vi "Property Finder (SubVI).vi"(8 "error in (no error)":errorcluster, 10 "Enum":enum16{"Read File", "Search for Property Name"}(ring), 11 "Property Name":string) -> (0 "error out":errorcluster, 3 "Property Value":string)   [LabVIEW 2018]
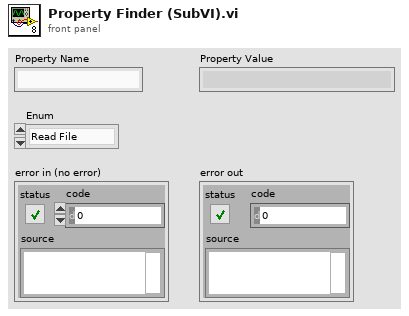
[diagram p1: front panel]
types:
  T1 = enum16{"open", "replace", "create", "open or create", "replace or create", "replace or create with confirmation"}
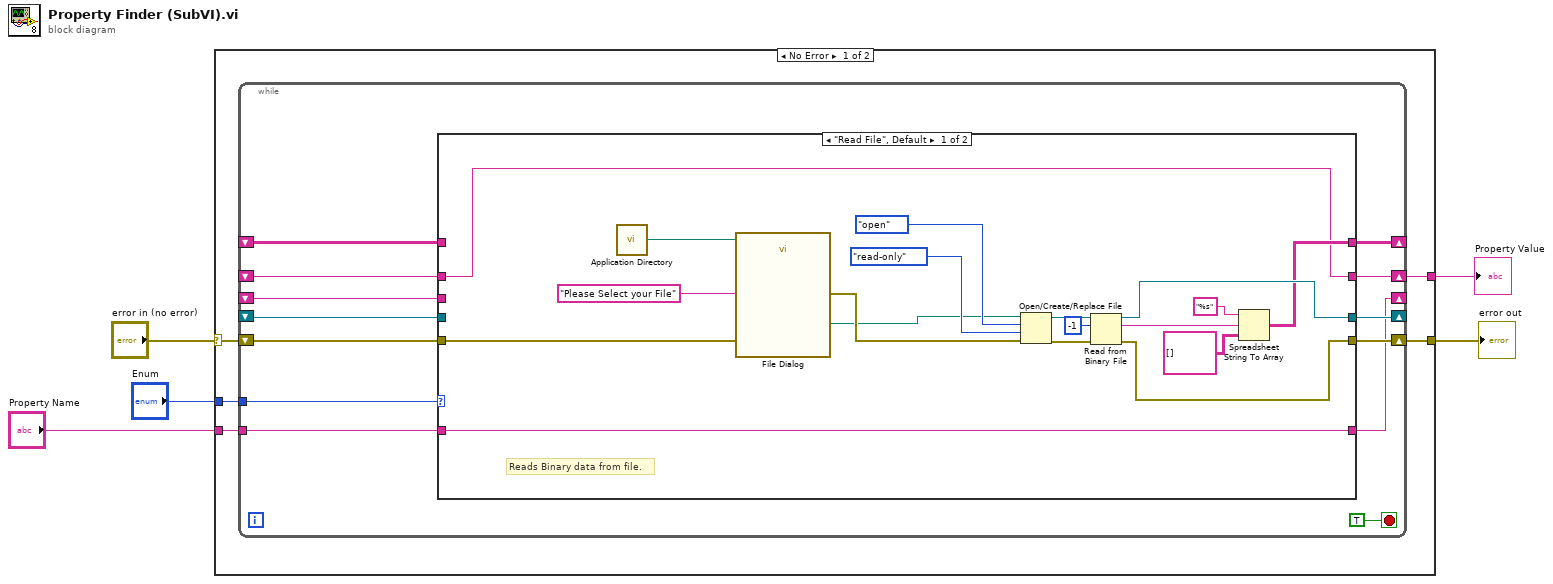
[diagram p0: block diagram]
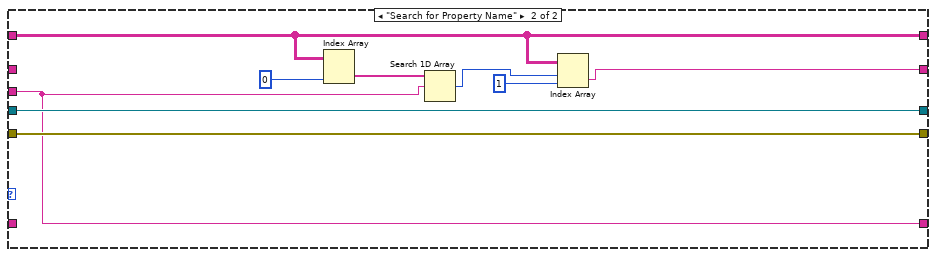
[diagram p2: hidden frame]
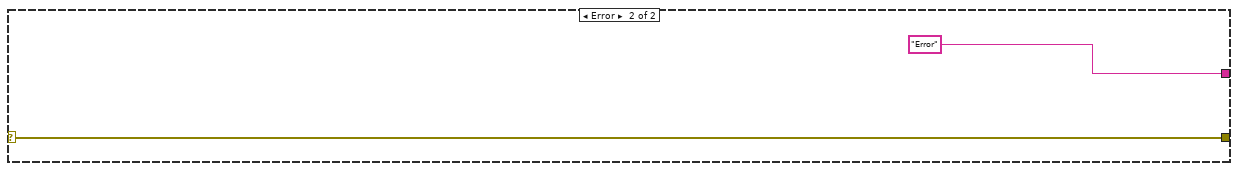
[diagram p3: hidden frame]
diagram:
  n1 = case shown="No Error" "error in (no error)" {
    selector: "error in (no error)" -> [w8 w52]
    tunnel: "Enum" -> [w10 _]
    tunnel: [w9 w52] -> w2
    tunnel: "Property Name" -> [w6 _]
    tunnel: [w7 "Error"] -> w5
    frame No Error {
      n2 = while {
        tunnel: w10 -> [w23]
        shift-right: [w21] -> w9
        shift-left: w8 -> [w20]
        shift-right: [w19] -> _
        shift-left: _ -> [w18]
        shift-right: [w16] -> _
        shift-left: _ -> [w17]
        shift-right: [w15] -> w7
        shift-left: _ -> [w14]
        shift-right: [w13] -> _
        shift-left: _ -> [w11]
        tunnel: w6 -> [w12]
        stop <- TRUE stop-if-true
        n3 = case shown="\"Read File\", Default" w23 {
          tunnel: [w29 w50] -> w21
          tunnel: w20 -> [w36 w50]
          tunnel: [w28 w49] -> w19
          tunnel: [w27 w46] -> w16
          tunnel: w18 -> [_ w49]
          tunnel: w17 -> [_ w46]
          tunnel: [w26 w43] -> w15
          tunnel: w14 -> [w26 _]
          tunnel: [w25 w42] -> w13
          tunnel: w12 -> [w25 _]
          tunnel: w11 -> [_ w42]
          frame "Read File", Default {
            # "Reads Binary data from file."
            n4 = call <vilib>:"Application Directory.vi"() -> ("Application Directory"=w24:path)
            n5 = call "File Dialog"("start path"=w24, "prompt"="Please Select your File", "error in"=w36) -> ("selected path"=w33:path, "error out"=w35:errorcluster)  [unwired: 9 in, 2 out]
            n6 = Open/Create/Replace File(file path (use dialog)=w33, error in=w35, operation (0:open)=T1."open", access (0:read/write)=enum16{"read/write", "read-only", "write-only"}."read-only") -> (refnum out=w39:refnum<file>, error out=w38:errorcluster)  [unwired: 2 in, 1 out]
            n7 = Read from Binary File(8:w38, 10:-1 ("count (1)"), 11:w39) -> (0:w29:errorcluster, 2:w30:string, 3:w28:refnum<file>)  [unwired: 3 in, 1 out]
            n8 = Spreadsheet String To Array(format string="%s", spreadsheet string=w30, array type (2D Dbl)=string[][] []) -> (array=w27:string[][])  [unwired: 1 in]
          }
          frame "Search for Property Name" {
            n9 = Index Array(array=w46, index (col)=0 ("disabled index (col)")) -> (element=w45:string[])  [unwired: 1 in]
            n10 = Search 1D Array(1D array=w45, element=w42) -> (index of element=w44:i32)  [unwired: 1 in]
            n11 = Index Array(array=w46, index (row)=w44, index (col)=1 ("disabled index (col)")) -> (element=w43:string)
          }
        }
      }
    }
    frame Error {
    }
  }
  "Property Value" <- w5
  "error out" <- w2
